vi "BK_PRECISION_XLN3640_set_voltage(SubVI).vi"(8 "Error In":errorcluster, 10 "voltage":string, 11 "Connect in":T1) -> (0 "error out":errorcluster, 3 "Connect out":T1)   [LabVIEW 2018]
uses:
  MOKO_LabViewLibrary/MokoLowLevel/MokoLowLovelControl/MLLC_ConnectCluster.ctl
  MOKO_LabViewLibrary/MokoLowLevel/MokoLowLovelControl/MLLC_InterfaceType.ctl
  MOKO_LabViewLibrary/MokoLowLevel/MokoLowLovelControl/MLLC_OpenedSession.ctl
  MOKO_LabViewLibrary/MokoLowLevel/MokoLowLovelControl/MLLC_InterfaceSettings.ctl
  MOKO_LabViewLibrary/MokoLowLevel/MokoLowLovelControl/MLLC_InterfaceKind.ctl
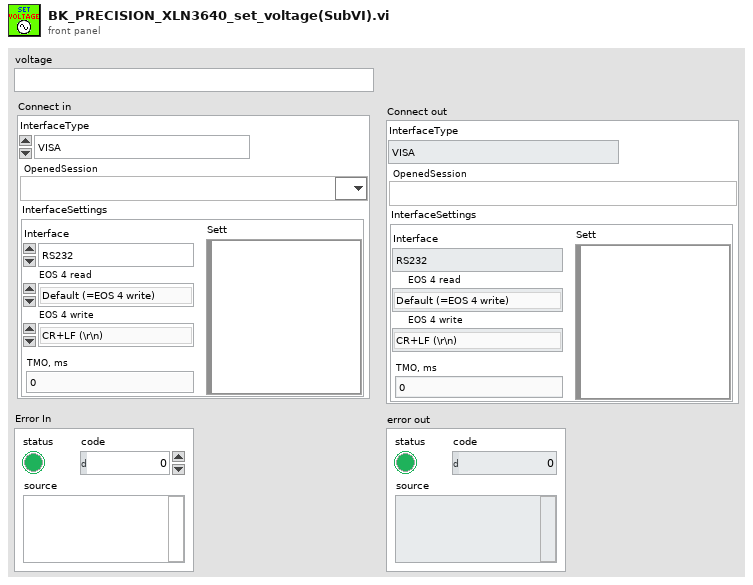
[diagram p1: front panel]
types:
  T1 = typedef "MLLC_ConnectCluster.ctl" = cluster{"InterfaceType":T2, "OpenedSession":T3, "InterfaceSettings":T4}
  T2 = typedef "MLLC_InterfaceType.ctl" = enum16{"VISA", "Prologix USB-GPIB"}
  T3 = typedef "MLLC_OpenedSession.ctl" = refnum<visa-resource-name>
  T4 = typedef "MLLC_InterfaceSettings.ctl" = cluster{"Interface":T5, "EOS 4 read":enum16{"Default (=EOS 4 write)", "CR (\\r)", "LF (\\n)", "None"}, "EOS 4 write":enum16{"CR+LF (\\r\\n)", "CR (\\r)", "LF (\\n)", "None"}, "TMO, ms":i32, "Sett":variant}
  T5 = typedef "MLLC_InterfaceKind.ctl" = enum16{"RS232", "GPIB", "USB", "Ethernet", "another"}
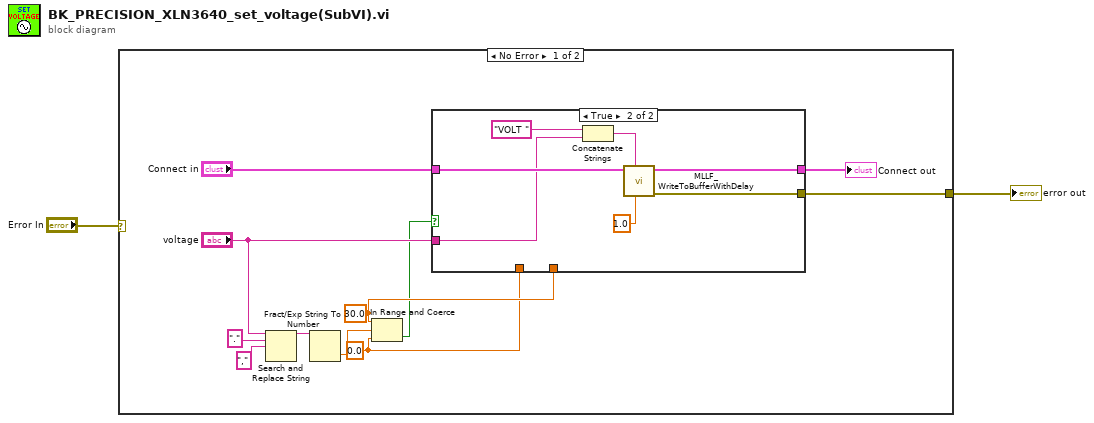
[diagram p0: block diagram]
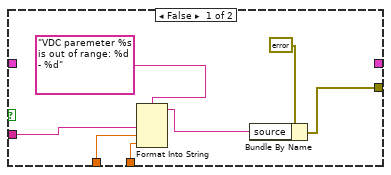
[diagram p2: hidden frame]
diagram:
  n1 = case shown="No Error" "Error In" {
    selector: "Error In" -> [_ w28]
    tunnel: [w13 w28] -> w2
    frame No Error {
      w12 = 30.0 ("upper limit")
      w11 = 0.0 ("lower limit")
      n2 = Search and Replace String(input string="voltage", search string="." ("substring (\"\")"), replace string="," ("replace string (\"\")")) -> (result string=w5:string)  [unwired: 5 in, 3 out]
      n3 = Fract/Exp String To Number(string=w5) -> (number=w8:dbl)  [unwired: 3 in, 1 out]
      n4 = In Range and Coerce(upper limit=w12, x=w8, lower limit=w11) -> (In Range?=w9:bool)  [unwired: 1 out]
      n5 = case shown="True" w9 {
        tunnel: "Connect in" -> [_ w27]
        tunnel: "voltage" -> [w18 w25]
        tunnel: [w19 w22] -> w13
        tunnel: w11 -> [w16 _]
        tunnel: w12 -> [w15 _]
        tunnel: [_ w21] -> w3
        frame False {
          n6 = Format Into String(format string="VDC paremeter %s is out of range: %d - %d", w18, w16, w15) -> (resulting string=w14:string)  [unwired: 2 in, 1 out]
          n7 = Bundle By Name(cluster=errorcluster {"status"=TRUE, "code"=400, "source"=""} ("error out"), "source"=w14) -> (w19:errorcluster)
        }
        frame True {
          n8 = Concatenate Strings("VOLT ", w25) -> (w23:string)
          n9 = call "MLLF_WriteToBufferWithDelay.vi"("Delay Time ( 0,05 s)"=1.0 ("Delay Time (s)"), "Command"=w23, "DriverConnect in"=w27) -> ("Error Out"=w22:errorcluster, "DriverConnect out"=w21:T1)  [unwired: 7 in]
        }
      }
      "Connect out" <- w3
    }
    frame Error {
    }
  }
  "error out" <- w2
